vi "Config.vi"(8 "error in (no error)":errorcluster, 10 "Setting":variant, 11 "Analog In in":refnum<class "Analog In.lvclass">) -> (0 "error out":errorcluster, 3 "Analog In out":refnum<class "Analog In.lvclass">)   [LabVIEW 2019, in "Hardware Abstration.lvlib" / "Analog In.lvclass"]
uses:
  Analog In.lvclass
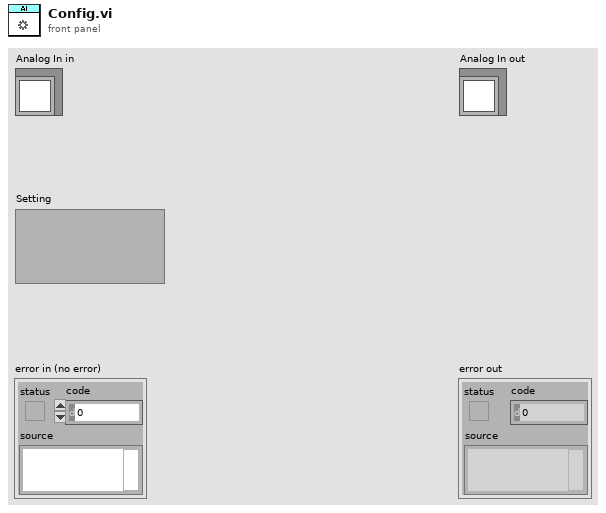
[diagram p1: front panel]
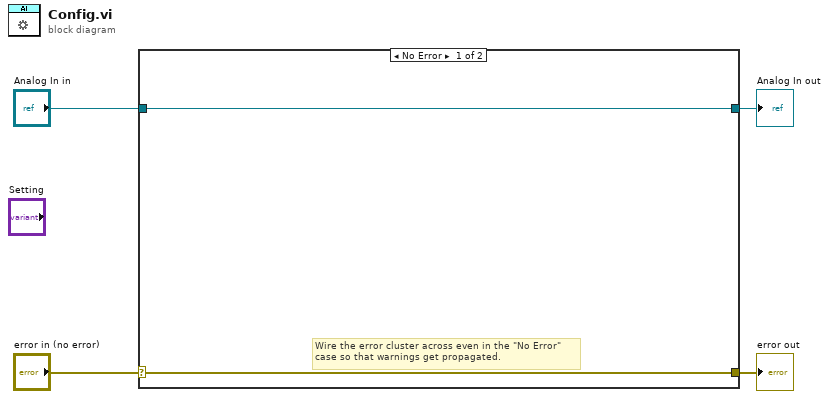
[diagram p0: block diagram]
diagram:
  n1 = case shown="No Error" "error in (no error)" {
    selector: "error in (no error)" -> [w5 w8]
    tunnel: [w5 w8] -> w3
    tunnel: [w6 w7] -> w1
    tunnel: "Analog In in" -> [w6 w7]
    frame No Error {
      # "Wire the error cluster across even in the \"No Error\"\ncase so that warnings get propagated."
    }
    frame Error {
    }
  }
  "error out" <- w3
  "Analog In out" <- w1
